vi "a_plus_b_cube.vi"() -> ()   [LabVIEW 2026]
panel:
  in  "b":dbl
  out "(a+b)^3":dbl
  in  "a":dbl
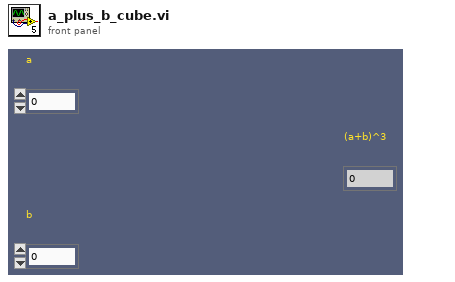
[diagram p1: front panel]
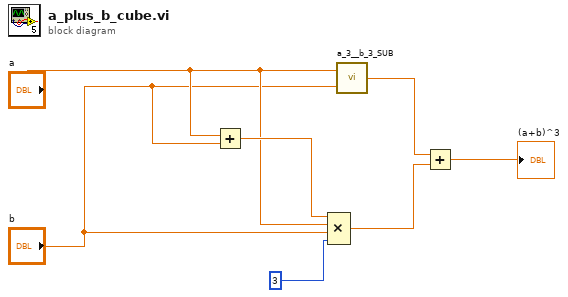
[diagram p0: block diagram]
diagram:
  n1 = Add(x="a", y="b") -> (x+y=w7:dbl)
  n2 = Compound Arithmetic op=MULTIPLY(w7, "a", "b", 3) -> (w3:dbl)
  n3 = call "a_3__b_3_SUB.vi"("b"="b", "a"="a") -> ("a^3+b^3"=w2:dbl)
  n4 = Add(x=w2, y=w3) -> (x+y=→"(a+b)^3":dbl)
